vi "Write Table Name.vi"(8 "error in (no error)":errorcluster, 10 "Table Name":string, 11 "SQLite configuration in":refnum<class "SQLite configuration.lvclass">) -> (0 "error out":errorcluster, 3 "SQLite configuration out":refnum<class "SQLite configuration.lvclass">)   [LabVIEW 2014, in "SQLite configuration.lvclass"]
uses:
  SQLite configuration.lvclass
  SQLite configuration.lvclass/SQLite configuration.ctl
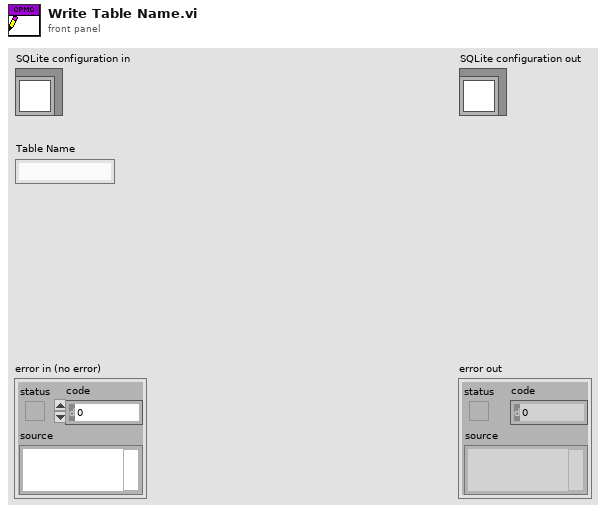
[diagram p1: front panel]
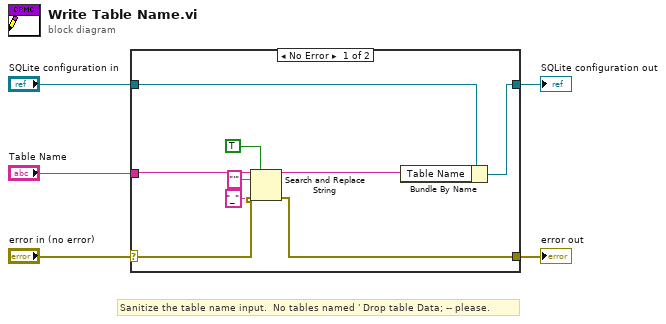
[diagram p0: block diagram]
diagram:
  # "Sanitize the table name input.  No tables named ' Drop table Data; -- please."
  n1 = case shown="No Error" "error in (no error)" {
    selector: "error in (no error)" -> [w9 w15]
    tunnel: [w8 w15] -> w4
    tunnel: [w13 w16] -> w2
    tunnel: "SQLite configuration in" -> [w14 w16]
    tunnel: "Table Name" -> [w11 _]
    frame No Error {
      n2 = Search and Replace String(replace all?=TRUE ("replace all? (F)"), input string=w11, search string="'", replace string="_" ("replace string (\"\")"), error in=w9) -> (result string=w10:string, error out=w8:errorcluster)  [unwired: 3 in, 2 out]
      n3 = Bundle By Name(cluster=w14, "Table Name"=w10) -> (w13:refnum<class "SQLite configuration.lvclass">)
    }
    frame Error {
    }
  }
  "error out" <- w4
  "SQLite configuration out" <- w2
